vi "averaging position values.vi"(3 "Beam sorted SUM":dbl[][](array[numeric]), 4 "Beam sorted Y":dbl[][](array[numeric]), 5 "Beam sorted X data":dbl[][](array[numeric])) -> (0 "SUM avg":dbl[](array[numeric]), 1 "Y avg":dbl[](array[numeric]), 2 "X avg":dbl[](array[numeric]))   [LabVIEW 2020]
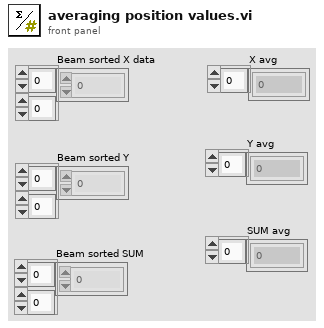
[diagram p1: front panel]
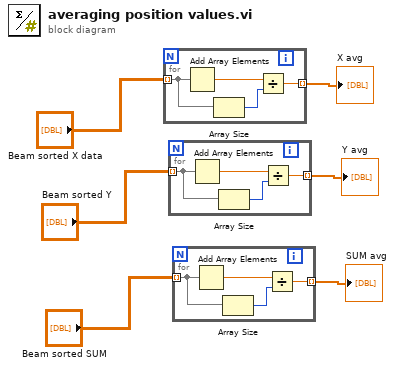
[diagram p0: block diagram]
diagram:
  n1 = for {
    tunnel: "Beam sorted X data" -> [w8] mode=indexing
    tunnel: [w7] -> w6 mode=indexing
    n2 = Add Array Elements(numeric array=w8) -> (sum=w10:dbl)
    n3 = Array Size(array=w8) -> (size(s)=w9:i32)
    n4 = Divide(x=w10, y=w9) -> (x/y=w7:dbl)
  }
  "X avg" <- w6
  n5 = for {
    tunnel: "Beam sorted Y" -> [w12] mode=indexing
    tunnel: [w11] -> w4 mode=indexing
    n6 = Add Array Elements(numeric array=w12) -> (sum=w14:dbl)
    n7 = Array Size(array=w12) -> (size(s)=w13:i32)
    n8 = Divide(x=w14, y=w13) -> (x/y=w11:dbl)
  }
  "Y avg" <- w4
  n9 = for {
    tunnel: "Beam sorted SUM" -> [w16] mode=indexing
    tunnel: [w15] -> w2 mode=indexing
    n10 = Add Array Elements(numeric array=w16) -> (sum=w18:dbl)
    n11 = Array Size(array=w16) -> (size(s)=w17:i32)
    n12 = Divide(x=w18, y=w17) -> (x/y=w15:dbl)
  }
  "SUM avg" <- w2
